vi "zadanie3.vi"() -> ()   [LabVIEW 2019]
uses:
  <vilib>/Analysis/2dsp.llb/Real FFT.vi
  <vilib>/measure/maspectr.llb/FFT Spectrum (Mag-Phase) for 1 Chan.vi
  <vilib>/Analysis/NI_AALPro.lvlib
  <vilib>/measure/NI_MAPro.lvlib
panel:
  out "Waveform Graph 4":cluster{"f0":dbl, "df":dbl, "magnitude":dbl[]}(graph)
  out "Waveform Graph 3":dbl[](graph)
  out "Waveform Graph 2":dbl[](graph)
  out "Hz":cluster{"X[Hz]":dbl, "\nY":dbl}
  out "Cursor difference":cluster{"X[s]":dbl, "Y[V]":dbl}
  out "Waveform Graph":cluster{dbl, dbl, "array type ":dbl[]}(graph)
  out "array":dbl[](array[numeric])
  out "read buffer":string
  in  "RUN":bool
  in  "stop":bool
  in  "byte count":u32
  in  "Sine Wave":T1={"Frequency [Hz]"=50.0, "Amplitude [V]"=2.0, "Offset [V]"=2.5}
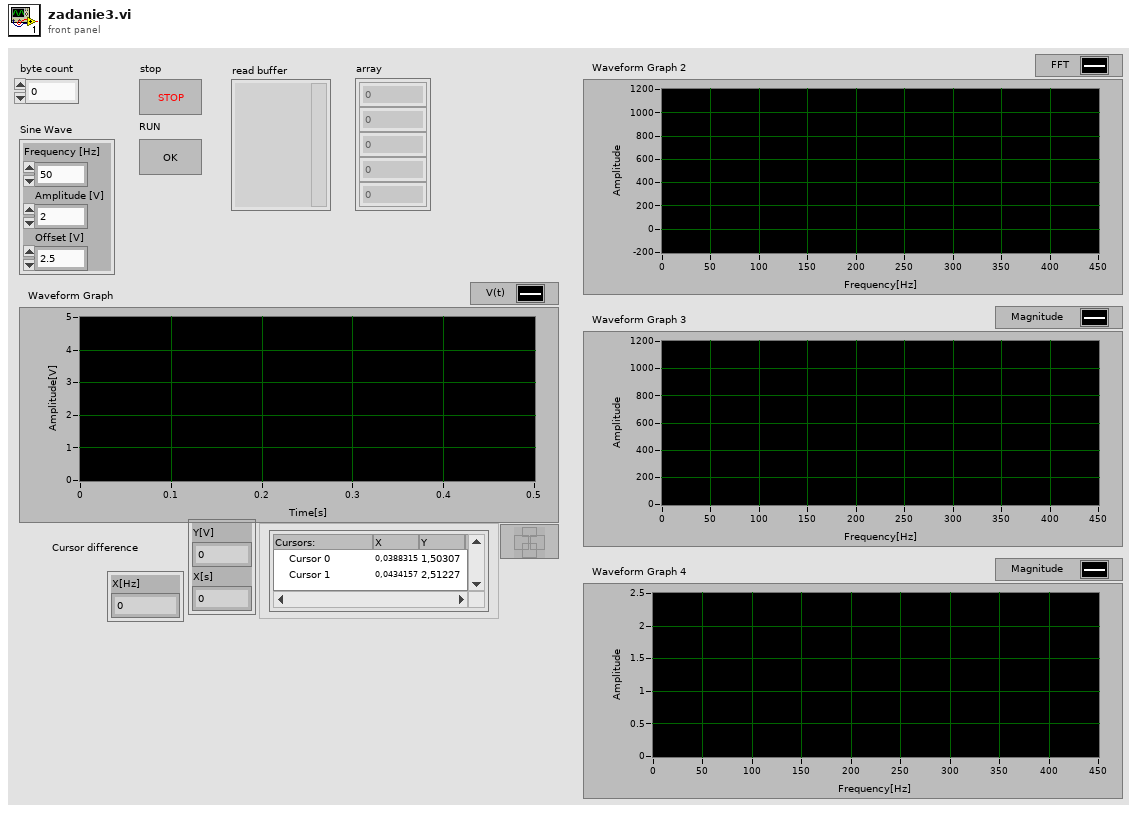
[diagram p1: front panel]
types:
  T1 = cluster{"Frequency [Hz]":dbl, "Amplitude [V]":dbl, "Offset [V]":dbl}
  T2 = typedef "LVCursorListTypeDef.ctl" = cluster{"Name":string, "Color":u32, "Style":u8, "Point Style":u8, "Name Visible":bool, "Allow Drag":bool, "Cursor Mode":u32, "Plot":i32, "Index":i32, "Position":cluster{"X":dbl, "Y":dbl}, "X Scale":u32, "Y Scale":u32, "Watch Plots":i32[], "Watch All Plots":bool, "Plot Area":i32, "Label Offset":cluster{"X":dbl, "Y":dbl}}[]
  T3 = cluster{"Name":string, "Color":u32, "Style":u8, "Point Style":u8, "Name Visible":bool, "Allow Drag":bool, "Cursor Mode":u32, "Plot":i32, "Index":i32, "Position":cluster{"X":dbl, "Y":dbl}, "X Scale":u32, "Y Scale":u32, "Watch Plots":i32[], "Watch All Plots":bool, "Plot Area":i32, "Label Offset":cluster{"X":dbl, "Y":dbl}}
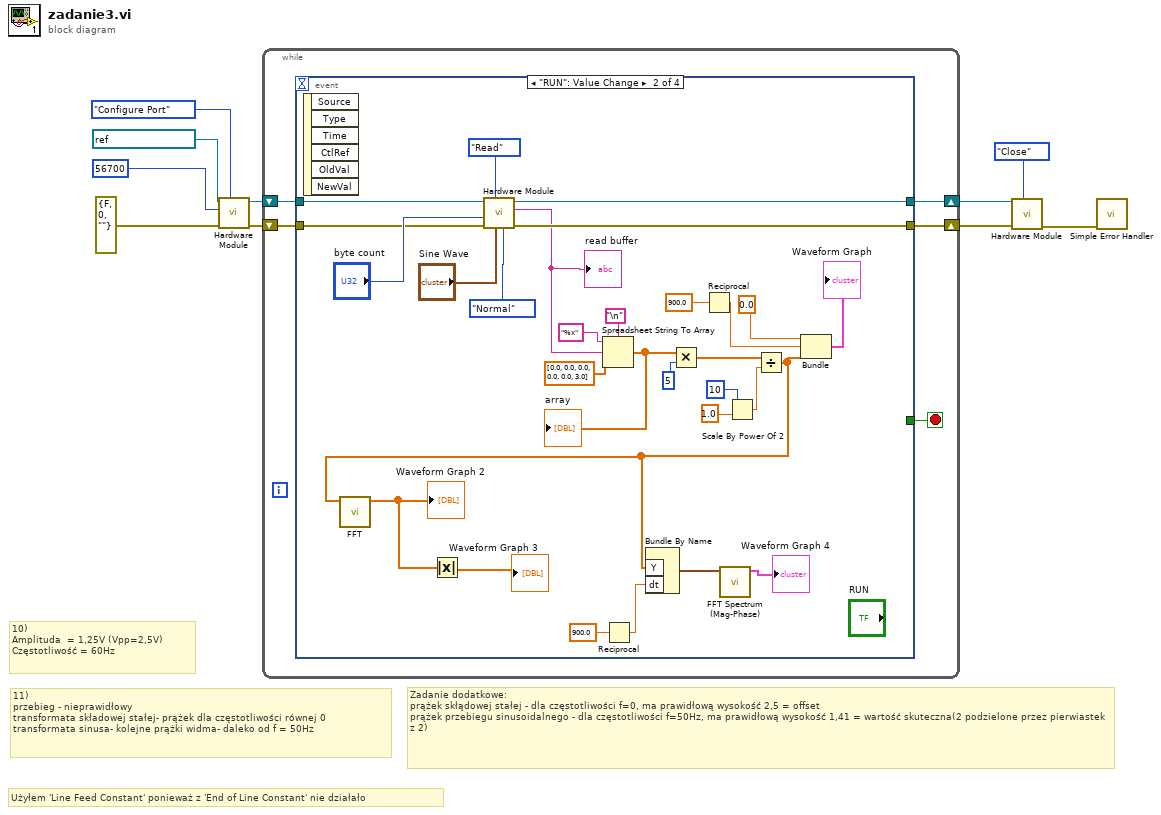
[diagram p0: block diagram]
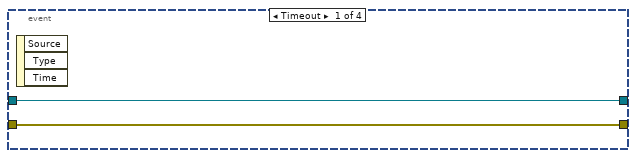
[diagram p2: hidden frame]
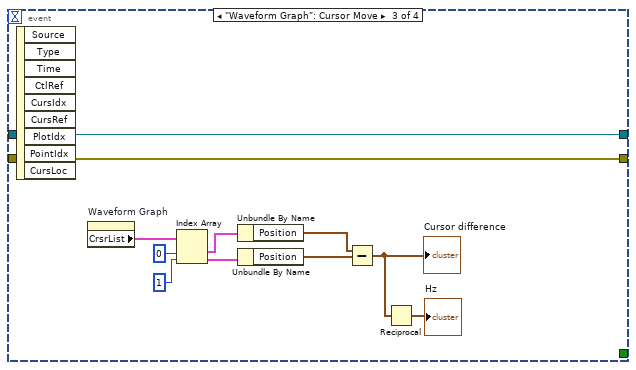
[diagram p3: hidden frame]
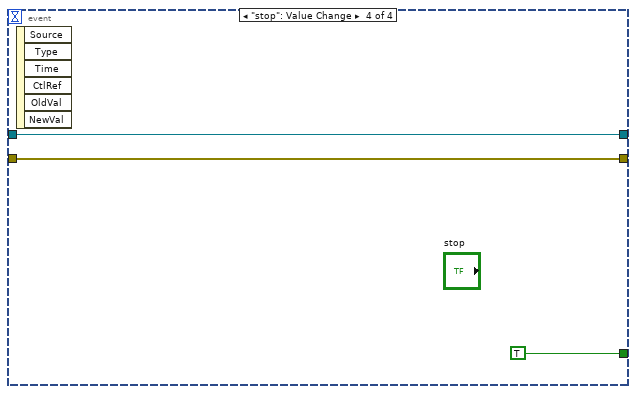
[diagram p4: hidden frame]
diagram:
  # "Zadanie dodatkowe:\nprążek skłądowej stałej - dla częstotliwości f=0, ma prawidłową wysokość 2,5 = offset\nprążek przebiegu sinusoidalnego - dla częstotliwości f=50Hz, ma prawidłową wysokość 1,41 = wartość skuteczna(2 podzielone przez pierwiastek z 2)"
  # "11)\nprzebieg - nieprawidłowy\ntransformata składowej stałej- prążek dla częstotliwości równej 0\ntransformata sinusa- kolejne prążki widma- daleko od f = 50Hz"
  # "10)\nAmplituda  = 1,25V (Vpp=2,5V)\nCzęstotliwość = 60Hz"
  # "Użyłem 'Line Feed Constant' ponieważ z 'End of Line Constant' nie działało"
  n1 = call "Hardware Module.vi"("State"=enum16{"Configure Port", "Read", "Close"}."Configure Port", "error in (no error)"=errorcluster {"status"=FALSE, "code"=0, "source"=""}, "baud rate (9600)"=u32 56700, "VISA resource name"=refnum<visa-resource-name> "VirtualDevice1") -> ("error out"=w7:errorcluster, "VISA resource name out"=w6:refnum<visa-resource-name>)  [unwired: 5 in, 1 out]
  n2 = while {
    shift-right: [w13] -> w5
    shift-left: w7 -> [w15]
    shift-right: [w12] -> w4
    shift-left: w6 -> [w14]
    stop <- w11 stop-if-true
    n3 = event shown="[1] \"RUN\": Value Change" {
      selector: _ -> [_ _ _ _]
      dyn-events: _ -> [_ _ _ _]
      timeout: _ -> [_ _ _ _]
      tunnel: w15 -> [w16 w39 w56 w59]
      tunnel: w14 -> [w17 w40 w57 w60]
      tunnel: [w16 w42 w56 w59] -> w13
      tunnel: [w17 w41 w57 w60] -> w12
      tunnel: [_ _ _ TRUE ("RUN")] -> w11
      event Timeout {
        n4 = event-data() -> ()  [unwired: 1 in, 3 out]
      }
      event "RUN": Value Change {
        n5 = event-data() -> ()  [unwired: 1 in, 6 out]
        n6 = call "Hardware Module.vi"("Mode"=enum16{"Normal", "Hidden"}."Normal", "Sine Wave"="Sine Wave", "State"=enum16{"Configure Port", "Read", "Close"}."Read", "error in (no error)"=w39, "byte count"="byte count", "VISA resource name"=w40) -> ("error out"=w42:errorcluster, "read buffer"=w35:string, "VISA resource name out"=w41:refnum<visa-resource-name>)  [unwired: 3 in]
        "read buffer" <- w35
        n7 = Spreadsheet String To Array(delimiter (Tab)="\n", format string="%x", spreadsheet string=w35, array type (2D Dbl)=dbl[] [0.0, 0.0, 0.0, 0.0, 0.0, 3.0] ("array type")) -> (array=w28:dbl[])
        "array" <- w28
        n8 = Reciprocal(x=900.0) -> (1/x=w20:dbl)
        n9 = Multiply(x=w28, y=i16 5 ("n")) -> (x*y=w26:dbl[])
        n10 = Reciprocal(x=900.0) -> (1/x=w33:dbl)
        n11 = Scale By Power Of 2(n=i16 10, x=1.0) -> (x*2^n=w25:dbl)
        n12 = Divide(x=w26, y=w25) -> (x/y=w18:dbl[])
        n13 = call-poly <vilib>:"FFT.vi"("X"=w18) -> ("FFT {X}"=w19:cdb[])  [unwired: 9 in, 1 out]
        "Waveform Graph 2" <- w19
        n14 = Absolute Value(x=w19) -> (abs(x)=→"Waveform Graph 3":dbl[])
        n15 = Bundle By Name("Y"=w18, "dt"=w20) -> (w23:waveform(dbl))  [unwired: 1 in]
        n16 = call-poly <vilib>:"FFT Spectrum (Mag-Phase).vi"("time signal"=w23) -> ("magnitude"=→"Waveform Graph 4":cluster{"f0":dbl, "df":dbl, "magnitude":dbl[]})  [unwired: 6 in, 4 out]
        n17 = Bundle(0.0, w33, w18) -> (→"Waveform Graph":cluster{dbl, dbl, dbl[]})  [unwired: 1 in]
      }
      event "Waveform Graph": Cursor Move {
        n18 = event-data() -> ()  [unwired: 1 in, 9 out]
        n19 = property on="Waveform Graph" class="WFGraph (strict)"() -> ("CrsrList"=w55:T2)  [unwired: 2 in, 2 out]
        n20 = Index Array(array=w55, index #1=0 ("index"), index #2=1 ("index")) -> (element #1=w52:T3, element #2=w51:T3)
        n21 = Unbundle By Name(w52) -> ("Position"=w50:cluster{"X":dbl, "Y":dbl})
        n22 = Unbundle By Name(w51) -> ("Position"=w49:cluster{"X":dbl, "Y":dbl})
        n23 = Subtract(x=w50, y=w49) -> (x-y=w48:cluster{"X":dbl, "Y":dbl})
        "Cursor difference" <- w48
        n24 = Reciprocal(x=w48) -> (1/x=→"Hz":cluster{"X":dbl, "Y":dbl})
      }
      event "stop": Value Change {
        n25 = event-data() -> ()  [unwired: 1 in, 6 out]
      }
    }
  }
  n26 = call "Hardware Module.vi"("State"=enum16{"Configure Port", "Read", "Close"}."Close", "error in (no error)"=w5, "VISA resource name"=w4) -> ("error out"=w1:errorcluster)  [unwired: 6 in, 2 out]
  n27 = call <vilib>:"Simple Error Handler.vi"("error in (no error)"=w1) -> ()  [unwired: 4 in, 5 out]
